vi "MergeSameRows.vi"(8 "error in (no error)":errorcluster, 11 "List in":refnum<class "List.lvclass">) -> (0 "error out":errorcluster, 3 "List out":refnum<class "List.lvclass">)   [LabVIEW 2015, in "List.lvclass"]
uses:
  List.lvclass
  List.lvclass/List.ctl
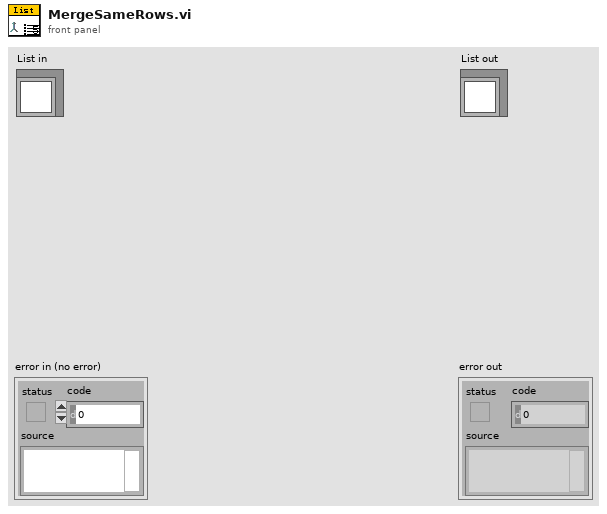
[diagram p1: front panel]
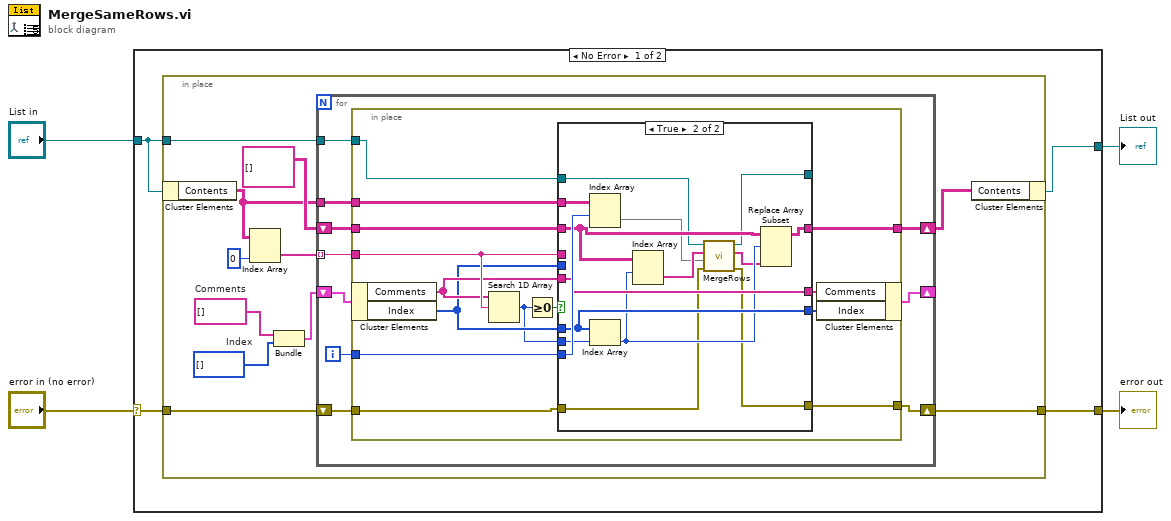
[diagram p0: block diagram]
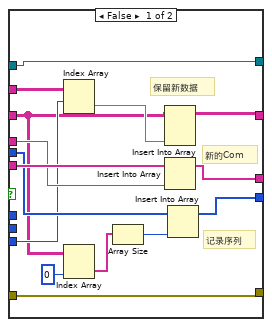
[diagram p2: hidden frame]
diagram:
  n1 = case shown="No Error" "error in (no error)" {
    selector: "error in (no error)" -> [w6 w75]
    tunnel: [w5 w75] -> w3
    tunnel: [w8 w74] -> w1
    tunnel: "List in" -> [w7 w74]
    frame No Error {
      n2 = in-place {
        in-place-border: w7 -> [w11]
        in-place-border: w6 -> [w10]
        in-place-border: [w9] -> w5
        w16 = i32[] []  # Index
        w17 = string[] []  # Comments
        n3 = in-place-cluster #1(w7) -> ("Contents"=w13:string[][])
        n4 = Index Array(array=w13, index (col)=0 ("disabled index (col)")) -> (element=w18:string[])  [unwired: 1 in]
        n5 = Bundle("Comments"=w17, "Index"=w16) -> (w15:cluster{"Comments":string[], "Index":i32[]})  [unwired: 1 in]
        n6 = for {
          tunnel: w18 -> [w29] mode=indexing
          shift-right: [w25] -> _
          shift-left: w15 -> [w27]
          shift-right: [w26] -> w12
          shift-left: string[][] [] ("Contents") -> [w28]
          tunnel: w13 -> [w24]
          tunnel: w11 -> [w22]
          shift-right: [w20] -> w9
          shift-left: w10 -> [w21]
          i -> [w23]
          n7 = in-place {
            in-place-border: w29 -> [w41]
            in-place-border: w28 -> [w42]
            in-place-border: [w37] -> w26
            in-place-border: w24 -> [w34]
            in-place-border: w23 -> [w33]
            in-place-border: w22 -> [w32]
            in-place-border: w21 -> [w31]
            in-place-border: [w30] -> w20
            n8 = in-place-cluster #2(w27) -> ("Comments"=w40:string[], "Index"=w36:i32[])
            n9 = Search 1D Array(1D array=w40, element=w41) -> (index of element=w35:i32)  [unwired: 1 in]
            n10 = Greater Or Equal To 0?(x=w35) -> (x >= 0?=w43:bool)
            n11 = case shown="True" w43 {
              tunnel: w42 -> [w46 w68]
              tunnel: w41 -> [w57 _]
              tunnel: w40 -> [w58 w69]
              tunnel: w36 -> [w56 _]
              tunnel: [w55 w69] -> w39
              tunnel: [w54 w70] -> w38
              tunnel: [w51 w66] -> w37
              tunnel: w36 -> [_ w70]
              tunnel: w35 -> [_ w71]
              tunnel: w34 -> [w53 w73]
              tunnel: w33 -> [w50 w72]
              tunnel: w32 -> [w47 w63]
              tunnel: [w47 w62] -> _
              tunnel: w31 -> [w48 w60]
              tunnel: [w48 w59] -> w30
              frame False {
                # "记录序列"
                # "新的Com"
                # "保留新数据"
                n12 = Index Array(array=w53, index (row)=w50) -> (element=w52:string[])  [unwired: 1 in]
                n13 = Index Array(array=w46, index (col)=0 ("disabled index (col)")) -> (element=w44:string[])  [unwired: 1 in]
                n14 = Array Size(array=w44) -> (size(s)=w49:i32)
                n15 = Insert Into Array(array=w46, new element=w52) -> (w51:string[][])  [unwired: 2 in]
                n16 = Insert Into Array(array=w58, new element=w57) -> (w55:string[])  [unwired: 1 in]
                n17 = Insert Into Array(array=w56, new element=w49) -> (w54:i32[])  [unwired: 1 in]
              }
              frame True {
                n18 = Index Array(array=w73, index (row)=w72) -> (element=w64:string[])  [unwired: 1 in]
                n19 = Index Array(array=w70, index=w71) -> (element=w67:i32)
                n20 = Index Array(array=w68, index (row)=w67) -> (element=w65:string[])  [unwired: 1 in]
                n21 = call-dynamic "MergeRows.vi"("error in (no error)"=w60, "RowContent(Slave)"=w64, "RowContent(Master)"=w65, "List.lvclass"=w63) -> ("error out"=w59:errorcluster, "NewContents"=w61:string[], "List.lvclass Out"=w62:refnum<class "List.lvclass">)  [unwired: 5 in]
                n22 = Replace Array Subset(array=w68, new element=w61, index (row)=w67) -> (w66:string[][])  [unwired: 1 in]
              }
            }
            n23 = in-place-cluster #2("Comments"=w39, "Index"=w38) -> (w25:cluster{"Comments":string[], "Index":i32[]})
          }
        }
        n24 = in-place-cluster #1("Contents"=w12) -> (w8:refnum<class "List.lvclass">)
      }
    }
    frame Error {
    }
  }
  "error out" <- w3
  "List out" <- w1
